vi "Read Core.vi"(8 "error in (no error)":errorcluster, 11 "WebView2.lvlib:WebView2 Control.lvclass":refnum<class "WebView2 QControl.lvclass">) -> (0 "error out":errorcluster, 2 "Webview2 Core":refnum<k24>, 3 "WebView2.lvlib:WebView2 Control.lvclass":refnum<class "WebView2 QControl.lvclass">)   [LabVIEW 2020, in "WebView2 QControl.lvlib" / "WebView2 QControl.lvclass"]
uses:
  WebView2 QControl.lvclass
  C:/Users/Simon/Documents/GitHub/LV-WebView2/Source/Libs/Microsoft.Web.WebView2.Core.dll
  Libs/Microsoft.Web.WebView2.Core.dll
  WebView2 QControl.lvclass/WebView2 QControl.ctl
  Webview2 Lib/WebView2 Control Object/WebView2 Control.lvclass
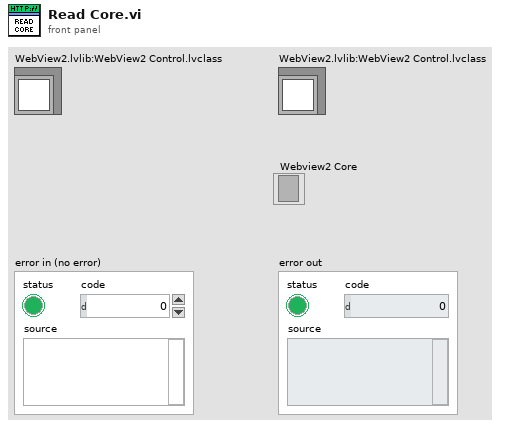
[diagram p1: front panel]
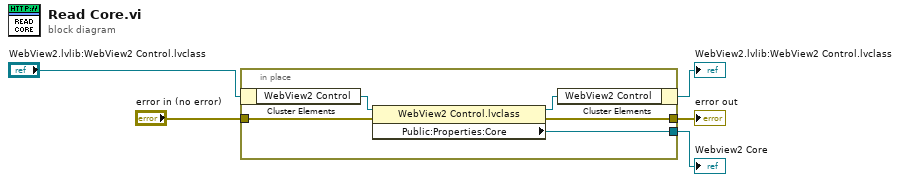
[diagram p0: block diagram]
diagram:
  n1 = in-place {
    in-place-border: "error in (no error)" -> [w10]
    in-place-border: [w9] -> w2
    in-place-border: [w6] -> w1
    n2 = in-place-cluster #1("WebView2.lvlib:WebView2 Control.lvclass") -> ("WebView2 Control"=w8:refnum<class "WebView2 Control.lvclass">)
    n3 = property class="WebView2 Control.lvclass"(reference=w8, error in=w10) -> (reference out=w7:refnum<class "WebView2 Control.lvclass">, error out=w9:errorcluster, "Public:Properties:Core"=w6:refnum<k24>)
    n4 = in-place-cluster #1("WebView2 Control"=w7) -> (→"WebView2.lvlib:WebView2 Control.lvclass":refnum<class "WebView2 QControl.lvclass">)
  }
  "error out" <- w2
  "Webview2 Core" <- w1
